vi "Release-status-notifiers.vi"(8 "error in (no error)":errorcluster, 11 "ModComm in":T1) -> (0 "error out":errorcluster, 3 "ModComm out":T1)   [LabVIEW 2013, in "Server.lvlib" / "Server.lvclass"]
uses:
  Server.lvclass
  Object-reference.ctl
  Server.lvclass/Server.ctl
  Read Exit.vi
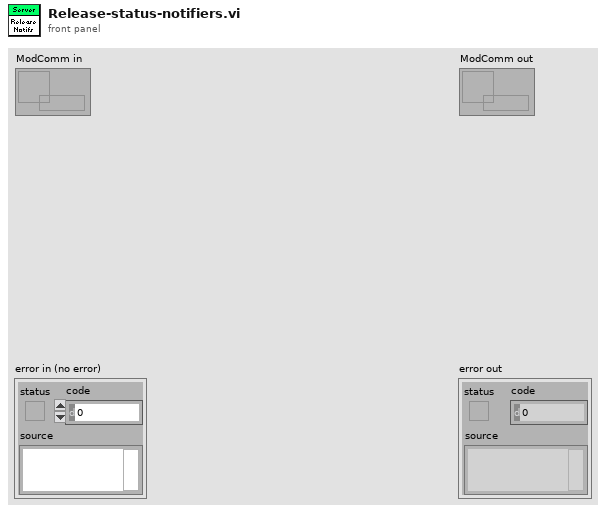
[diagram p1: front panel]
types:
  T1 = typedef "Server.lvlib/Server.lvclass/Object-reference.ctl" = refnum<data-value>
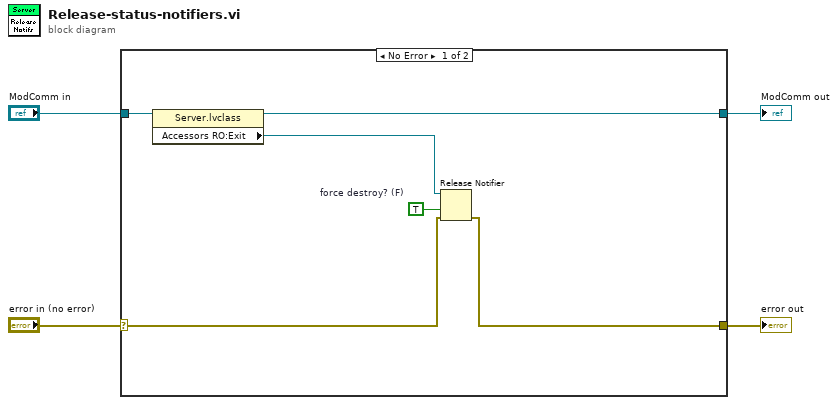
[diagram p0: block diagram]
diagram:
  n1 = case shown="No Error" "error in (no error)" {
    selector: "error in (no error)" -> [w7 w12]
    tunnel: [w6 w12] -> w3
    tunnel: [w9 w11] -> w1
    tunnel: "ModComm in" -> [w10 w11]
    frame No Error {
      w5 = TRUE  # force destroy? (F)
      n2 = property class="Server.lvclass"(reference=w10) -> (reference out=w9:T1, "Accessors RO:Exit"=w8:refnum<notifier>)  [unwired: 1 in, 1 out]
      n3 = Release Notifier(notifier=w8, force destroy? (F)=w5, error in (no error)=w7) -> (error out=w6:errorcluster)  [unwired: 2 out]
    }
    frame Error {
    }
  }
  "error out" <- w3
  "ModComm out" <- w1
